vi "Get URL Config.vi"(8 "error in (no error)":errorcluster, 11 "Plugin Model in":refnum<class "Plugin Configuration.lvclass">) -> (0 "error out":errorcluster, 2 "url config":T1, 3 "Plugin Model out":refnum<class "Plugin Configuration.lvclass">)   [LabVIEW 2016, in "Plugin Configuration.lvclass"]
uses:
  Plugin Configuration.lvclass
  Typedefs/Plugin Configuration.Typedef.URL Configuration.ctl
  Plugin Configuration.lvclass/Plugin Configuration.ctl
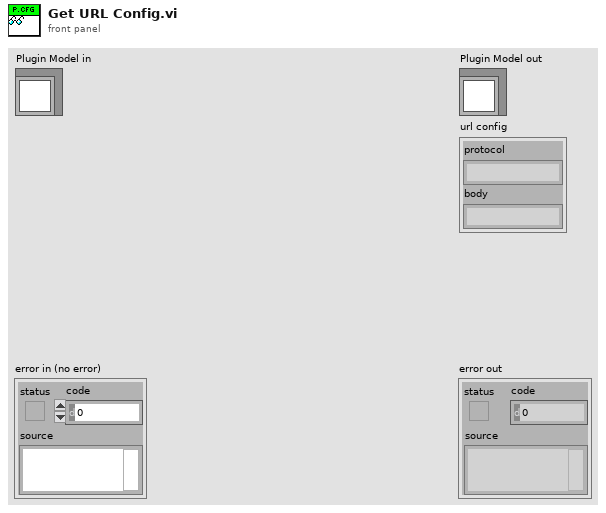
[diagram p1: front panel]
types:
  T1 = typedef "Plugin Configuration.lvclass/Plugin Configuration.Typedef.URL Configuration.ctl" = cluster{"protocol":string, "body":string}
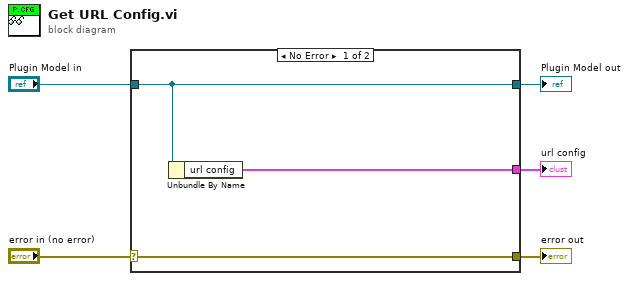
[diagram p0: block diagram]
diagram:
  n1 = case shown="No Error" "error in (no error)" {
    selector: "error in (no error)" -> [w8 w9]
    tunnel: [w8 w9] -> w4
    tunnel: [w7 w10] -> w2
    tunnel: "Plugin Model in" -> [w7 w10]
    tunnel: [w6 _] -> w1
    frame No Error {
      n2 = Unbundle By Name(w7) -> ("url config"=w6:T1)
    }
    frame Error {
    }
  }
  "error out" <- w4
  "Plugin Model out" <- w2
  "url config" <- w1
